vi "Trigger Actuator.vi"(5 "Time to wait":i32=999, 7 "error in":errorcluster, 8 "Target":i16, 9 "Actuator name":string, 10 "UTP IO Session in":T1) -> (0 "error out":errorcluster, 1 "ExpiredTimeToWait?":bool, 2 "Actuator was Ready?":bool=TRUE, 3 "UTP IO Session out":T1)   [LabVIEW 2023, in "Actuators.lvlib"]
doc: "Target 100 - Home position\nTarget 101 - Work position\nExpiredTimeToWait? => Rising/Falling edge wasn't detected\nThis VI will perform actuator action, if actutor is Ready (No errors)\nReading period is 10ms"
uses:
  Actuators.lvlib
  <vilib>/Noffz/UTP IO/UTP IO Library/Typedefs/Session Handle.ctl
  <vilib>/Noffz/UTP IO/UTP IO Library/UTP IO Pool Session.lvclass
  <vilib>/Noffz/UTP IO/UTP IO Library/methods/poly/plc/Write PLC Variable (I16).vi
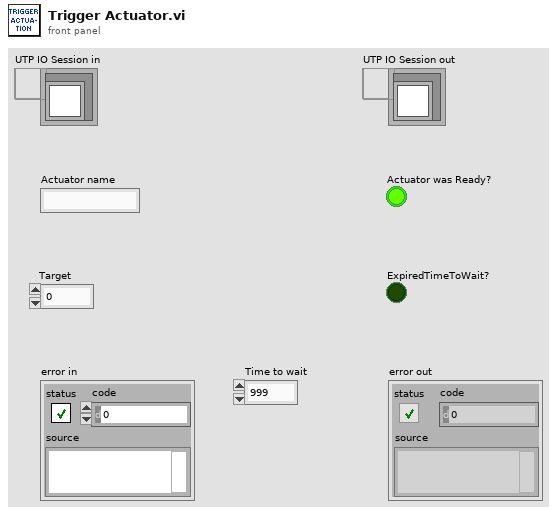
[diagram p1: front panel]
types:
  T1 = typedef "UTP IO Library.lvlib/UTP IO Pool Session.lvclass/Session Handle.ctl" = refnum<data-value>
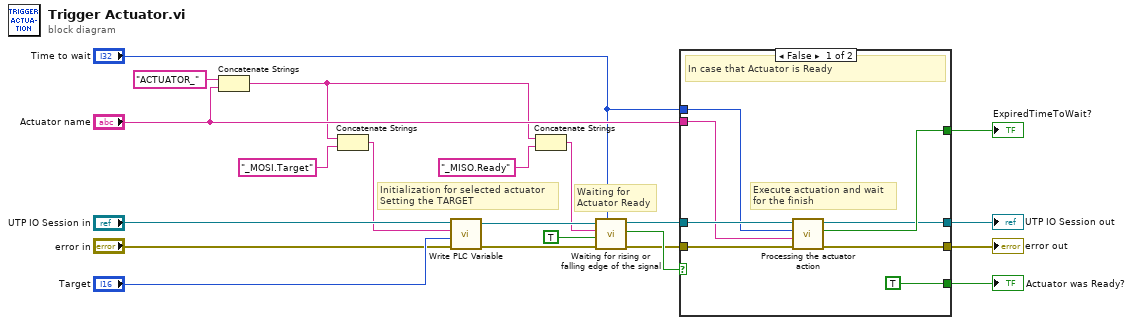
[diagram p0: block diagram]
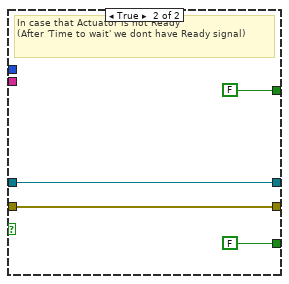
[diagram p2: hidden frame]
diagram:
  # "Waiting for \nActuator Ready"
  # "Initialization for selected actuator\nSetting the TARGET"
  n1 = Concatenate Strings("ACTUATOR_" ("string"), "Actuator name") -> (w5:string)
  n2 = Concatenate Strings(w5, "_MOSI.Target" ("string")) -> (w17:string)
  n3 = call-poly <vilib>:"Write PLC Variable.vi"("error in (no error)"="error in", "value"="Target", "variable name"=w17, "UTP IO Session in"="UTP IO Session in") -> ("error out"=w16:errorcluster, "UTP IO Session out"=w19:T1)  [unwired: 6 in]
  n4 = Concatenate Strings(w5, "_MISO.Ready" ("string")) -> (w3:string)
  n5 = call "Waiting for rising or falling edge of the signal.vi"("Time to wait"="Time to wait", "error in"=w16, "Rising/Falling edge"=TRUE, "Variable name"=w3, "UTP IO Session in"=w19) -> ("error out"=w11:errorcluster, "ExpiredTimeToWait?"=w12:bool, "UTP IO Session out"=w13:T1)  [unwired: 4 in]
  n6 = case shown="False" w12 {
    tunnel: [TRUE ("Elapsed30s?") FALSE ("Elapsed30s?")] -> w14
    tunnel: w13 -> [w28 w32]
    tunnel: "Actuator name" -> [w27 _]
    tunnel: w11 -> [w26 w31]
    tunnel: [w25 FALSE ("Elapsed 10s")] -> w10
    tunnel: [w24 w32] -> w8
    tunnel: [w23 w31] -> w7
    tunnel: "Time to wait" -> [w22 _]
    frame False {
      # "Execute actuation and wait \nfor the finish"
      # "In case that Actuator is Ready"
      n7 = call "Processing the actuator action.vi"("error in (no error)"=w26, "Actuator Name"=w27, "Time to wait"=w22, "UTP IO Session in"=w28) -> ("error out"=w23:errorcluster, "Elapsed TimeToWait?"=w25:bool, "UTP IO Session out"=w24:T1)  [unwired: 4 in]
    }
    frame True {
      # "In case that Actuator is not Ready \n(After 'Time to wait' we dont have Ready signal)"
    }
  }
  "Actuator was Ready?" <- w14
  "ExpiredTimeToWait?" <- w10
  "UTP IO Session out" <- w8
  "error out" <- w7
